vi "Read MAP DVR.vi"(8 "error in (no error)":errorcluster, 11 "Exe Write Main in":refnum<class "Exe Write Main.lvclass">) -> (0 "error out":errorcluster, 2 "MAP DVR":refnum<data-value>, 3 "Exe Write Main out":refnum<class "Exe Write Main.lvclass">)   [LabVIEW 2014, in "Controller.lvlib" / "Exe Write Main.lvclass"]
uses:
  Exe Write Main.lvclass
  Exe Write Main.lvclass/Exe Write Main.ctl
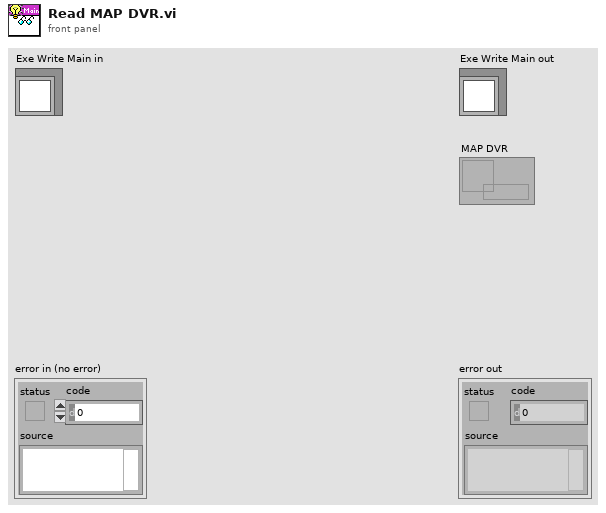
[diagram p1: front panel]
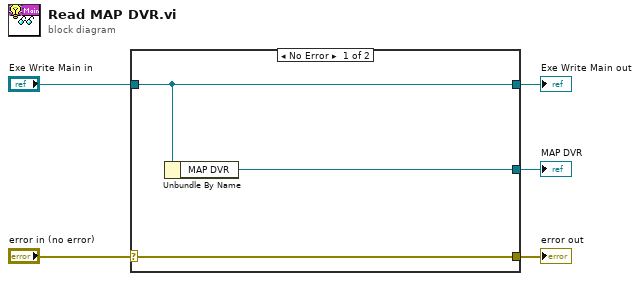
[diagram p0: block diagram]
diagram:
  n1 = case shown="No Error" "error in (no error)" {
    selector: "error in (no error)" -> [w8 w9]
    tunnel: [w8 w9] -> w4
    tunnel: [w7 w10] -> w2
    tunnel: "Exe Write Main in" -> [w7 w10]
    tunnel: [w6 _] -> w1
    frame No Error {
      n2 = Unbundle By Name(w7) -> ("MAP DVR"=w6:refnum<data-value>)
    }
    frame Error {
    }
  }
  "error out" <- w4
  "Exe Write Main out" <- w2
  "MAP DVR" <- w1
